vi "FIR Filter for N Chan.vi"(4 "optional FIR filter specifications":T2={"PB Gain"=-3.0, "SB Gain"=-60.0, "Scale"=TRUE, "Window"=enum."Flat Top"} {"SB Gain" format="%.2p"; "PB Gain" format="%.2p"}, 6 "FIR filter specifications":T3={"Topology"=enum."Off", "Type"=enum."Lowpass", "#Taps"=50, "Lower PB"=100.0, "Upper PB"=0.0, "Lower SB"=200.0, "Upper SB"=0.0} {"Lower SB" format="%0.2p"; "Upper SB" format="%0.2p"; "Lower PB" format="%0.2p"; "Upper PB" format="%0.2p"}, 7 "reset filters":bool, 8 "error in (no error)":errorcluster, 11 "signal(s) in":waveform(dbl)[](array[waveform])) -> (0 "error out":errorcluster, 2 "filter information":T1 {"phase H(w)"."df" format="%.2p"; "phase H(w)"."f0" format="%.2p"; "phase H(w)"."Phase H(w)" format="%.2p"; "magnitude H(w)"."df" format="%.2p"; "magnitude H(w)"."f0" format="%.2p"; "magnitude H(w)"."Mag H(w)" format="%.2p"}, 3 "signal(s) out":waveform(dbl)[](array[waveform]))   [LabVIEW 2020, in "NI_MAPro.lvlib"]
doc: "Filters signals in either single or multiple waveforms. If you are filtering multiple waveforms, the VI maintains separate filter states for each waveform. The data types you wire to the <B>signal in</B> and <B>FIR filter specifications</B> inputs determine the polymorphic instance to use."
uses:
  NI_MAPro.lvlib
  NI_MABase.lvlib
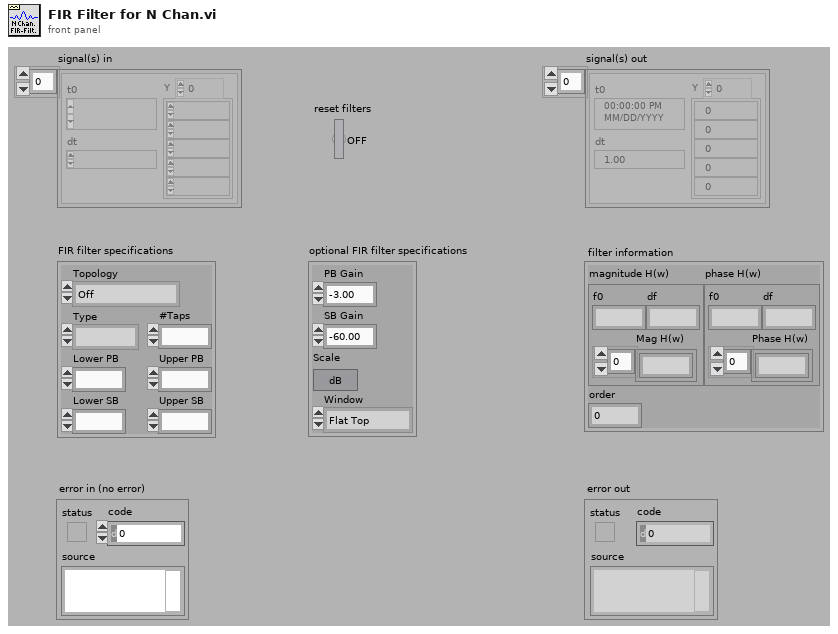
[diagram p1: front panel]
types:
  T1 = cluster{"magnitude H(w)":cluster{"f0":dbl, "df":dbl, "Mag H(w)":dbl[]}, "phase H(w)":cluster{"f0":dbl, "df":dbl, "Phase H(w)":dbl[]}, "order":i32}
  T2 = cluster{"PB Gain":dbl, "SB Gain":dbl, "Scale":bool, "Window":enum16{"None", "Hanning", "Hamming", "Triangular", "Blackman", "Exact Blackman", "Blackman-Harris", "Kaiser-Bessel", "Flat Top"}}
  T3 = cluster{"Topology":enum16{"Off", "FIR by Specification", "Equi-ripple FIR", "Windowed FIR"}, "Type":enum16{"Lowpass", "Highpass", "Bandpass", "Bandstop"}, "#Taps":i32, "Lower PB":dbl, "Upper PB":dbl, "Lower SB":dbl, "Upper SB":dbl}
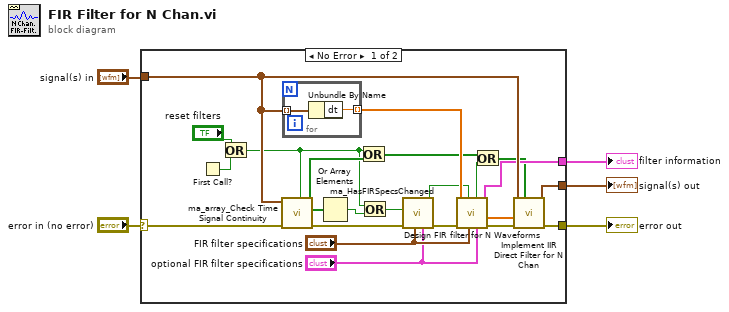
[diagram p0: block diagram]
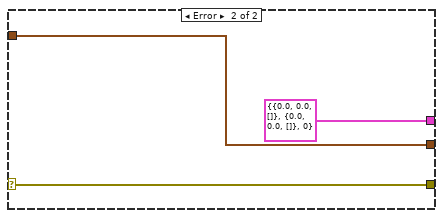
[diagram p2: hidden frame]
diagram:
  n1 = case shown="No Error" "error in (no error)" {
    selector: "error in (no error)" -> [w25 w32]
    tunnel: [w28 w32] -> w5
    tunnel: [w27 w33] -> w4
    tunnel: "signal(s) in" -> [w26 w33]
    tunnel: [w24 T1 {"magnitude H(w)"={"f0"=0.0, "df"=0.0, "Mag H(w)"=[]}, "phase H(w)"={"f0"=0.0, "df"=0.0, "Phase H(w)"=[]}, "order"=0} ("filter information")] -> w2
    frame No Error {
      n2 = First Call?() -> (First Call?: T/F=w9:bool)
      n3 = Or(x="reset filters", y=w9) -> (x .or. y?=w6:bool)
      n4 = call "ma_array_Check Time Signal Continuity.vi"("Ignore input time stamp"=w6, "error in (no error)"=w25, "waveforms"=w26) -> ("error out"=w16:errorcluster, "dt changed"=w15:bool[], "t0 changed"=w12:bool[])  [unwired: 5 in, 1 out]
      n5 = for {
        tunnel: w26 -> [w30] mode=indexing
        tunnel: [w29] -> w21 mode=indexing
        n6 = Unbundle By Name(w30) -> ("dt"=w29:dbl)
      }
      n7 = Or Array Elements(Boolean array=w15) -> (logical OR=w13:bool)
      n8 = Or(x=w6, y=w12) -> (x .or. y?=w11:bool[])
      n9 = Or(x=w6, y=w13) -> (x .or. y?=w14:bool)
      n10 = call "ma_HasFIRSpecsChanged.vi"("optional FIR filter specifications"="optional FIR filter specifications", "FIR Filter Specifications"="FIR filter specifications", "error in (no error)"=w16, "redesign filter"=w14) -> ("error out"=w18:errorcluster, "ValsDifferent?"=w17:bool)  [unwired: 6 in]
      n11 = call "Design FIR filter for N Waveforms.vi"("optional FIR filter specifications"="optional FIR filter specifications", "FIR filter specifications"="FIR filter specifications", "redesign filter"=w17, "error in"=w18, "arrdt"=w21) -> ("error out"=w23:errorcluster, "forward coefficients"=w22:dbl[], "filter information"=w24:T1, "reset filters"=w19:bool)  [unwired: 3 in]
      n12 = Or(x=w11, y=w19) -> (x .or. y?=w20:bool[])
      n13 = call "Implement IIR Direct Filter for N Chan.vi"("reset Filters"=w20, "error in (no error)"=w23, "Forward Coefficients"=w22, "arrWaveforms In"=w26) -> ("error out"=w28:errorcluster, "arrWaveforms Out"=w27:waveform(dbl)[])  [unwired: 6 in]
    }
    frame Error {
    }
  }
  "error out" <- w5
  "signal(s) out" <- w4
  "filter information" <- w2
